vi "find readout time.vi"(8 "error in (no error)":errorcluster, 11 "Simulated_CCD_Camera in":refnum<class "Sim_Ixon_Ultra.lvclass">) -> (0 "error out":errorcluster, 3 "Simulated_CCD_Camera out":refnum<class "Sim_Ixon_Ultra.lvclass">)   [LabVIEW 2018, in "Sim_Ixon_Ultra.lvclass"]
doc: "Find the readout time as a function of the operation mode of the CCD.\n\nThis value is used to determine the minimum exposure time allowed by ACS, that is the readout time plus 10 % of this value. This procedure is related to the functioning of the frame transfer mode of the CCD and it prevents the misuse of the exposure time."
uses:
  Sim_Ixon_Ultra.lvclass
  C:/Users/Denis/Desktop/S4ACS/S4ACS/Sim_CCD/Sim_CCD.lvclass
  Sim_Ixon_Ultra.lvclass/Sim_Ixon_Ultra.ctl
  <vilib>/Utility/file.llb/Read Delimited Spreadsheet (DBL).vi
  Sim_CCD/Sim_CCD.lvclass
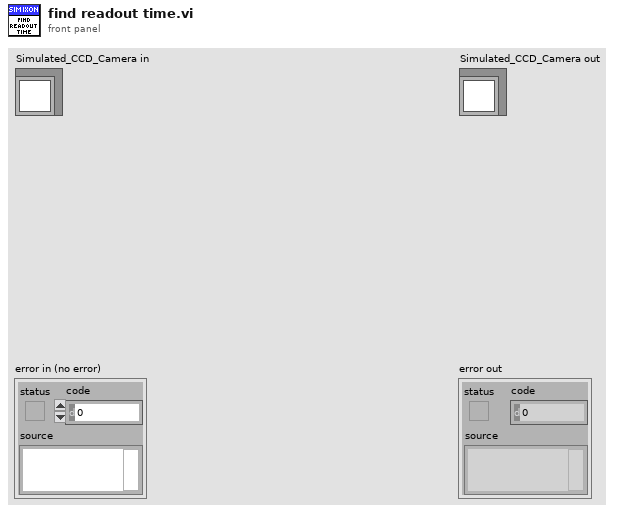
[diagram p1: front panel]
types:
  T1 = cluster{"PREAMP":u16, "READOUT_RATE":u16, "VERTICAL_SHIFT_SPEED":u16, "READ_MODE":u16, "VERTICAL_CLOCK_VOLTAGE":u16, "ACQUISITION_MODE":u16, "AD_CHANNEL":u16, "SHUTTER_TTL":u16, "SHUTTER_OPENING_TIME":u16, "SHUTTER_CLOSING_TIME":u16, "SHUTTER_MODE":u16, "TRIGGER_MODE":u16, "VBIN":u16, "INITIAL_LINE":u16, "INITIAL_COLUMN":u16, "FINAL_LINE":u16, "FINAL_COLUMN":u16, "HBIN":u16}
  T2 = typedef "LVDateTimeRec.ctl" = cluster{"fractional second":dbl, "second":i32, "minute":i32, "hour":i32, "day of month":i32, "month":i32, "year":i32, "day of week":i32, "day of year":i32, "DST":i32}
  T3 = cluster{"Time Acq Started":u32, "Image delay":u64, "Last update - CCD config":timestamp, "SYSTEMTIME":T2, "Readout time":dbl, "Time acq finished":u32, "effective exptime":dbl}
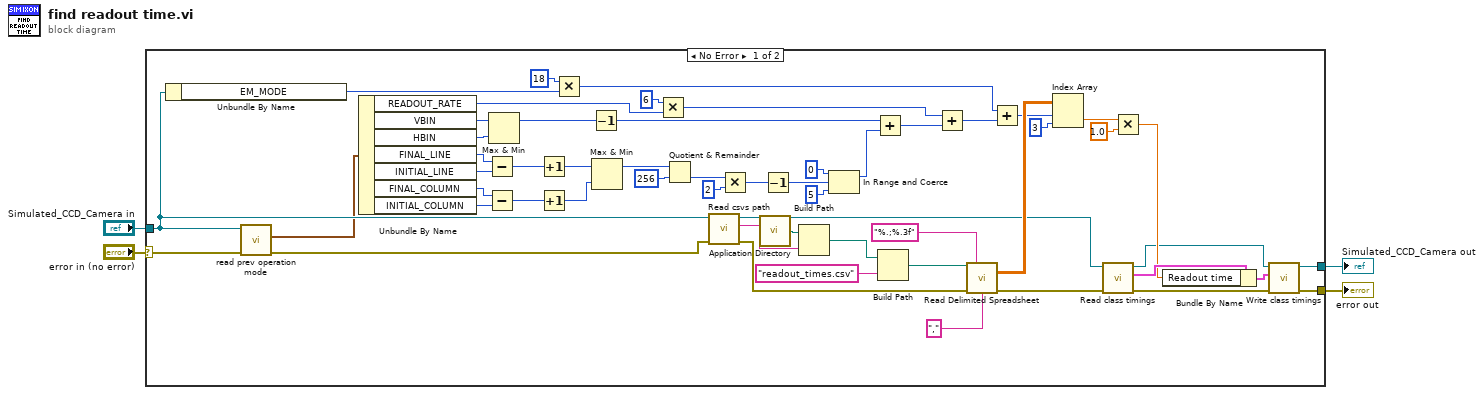
[diagram p0: block diagram]
diagram:
  n1 = case shown="No Error" "error in (no error)" {
    selector: "error in (no error)" -> [w7 w61]
    tunnel: [w19 w61] -> w3
    tunnel: [w21 w60] -> w1
    tunnel: "Simulated_CCD_Camera in" -> [w16 w60]
    frame No Error {
      n2 = Unbundle By Name(w16) -> ("EM_MODE"=w46:u16)
      n3 = call "read prev operation mode.vi"("error in (no error)"=w7, "Simulated_CCD_Camera in"=w16) -> ("error out"=w6:errorcluster, "prev operation mode"=w15:T1)  [unwired: 7 in, 1 out]
      n4 = Unbundle By Name(w15) -> ("READOUT_RATE"=w14:u16, "VBIN"=w13:u16, "HBIN"=w12:u16, "FINAL_LINE"=w11:u16, "INITIAL_LINE"=w10:u16, "FINAL_COLUMN"=w9:u16, "INITIAL_COLUMN"=w8:u16)
      n5 = Subtract(x=w11, y=w10) -> (x-y=w57:u16)
      n6 = Subtract(x=w9, y=w8) -> (x-y=w56:u16)
      n7 = Max & Min(x=w13, y=w12) -> (max(x,y)=w51:u16)  [unwired: 1 out]
      n8 = Increment(x=w57) -> (x+1=w55:u16)
      n9 = Increment(x=w56) -> (x+1=w54:u16)
      n10 = Multiply(x=u16 18, y=w46) -> (x*y=w43:u16)
      n11 = Decrement(x=w51) -> (x-1=w50:u16)
      n12 = Max & Min(x=w55, y=w54) -> (max(x,y)=w52:u16)  [unwired: 1 out]
      n13 = Multiply(x=u16 6, y=w14) -> (x*y=w47:u16)
      n14 = Quotient & Remainder(x=w52, y=u16 256) -> (floor(x/y)=w37:u16)  [unwired: 1 out]
      n15 = call "Read csvs path.vi"("error in (no error)"=w6, "Simulated Camera in"=w16) -> ("error out"=w26:errorcluster, "csvs path"=w5:string, "Simulated Camera out"=w18:refnum<class "Sim_Ixon_Ultra.lvclass">)  [unwired: 7 in]
      n16 = Multiply(x=w37, y=u16 2 ("x")) -> (x*y=w38:u16)
      n17 = call <vilib>:"Application Directory.vi"() -> ("Application Directory"=w58:path)
      n18 = Decrement(x=w38) -> (x-1=w36:u16)
      n19 = Build Path(base path=w58, name or relative path=w5) -> (appended path=w30:path)
      n20 = In Range and Coerce(upper limit=u16 0, x=w36, lower limit=u16 5 ("upper limit")) -> (coerced(x)=w33:u16)  [unwired: 1 out]
      n21 = Add(x=w50, y=w33) -> (x+y=w48:u16)
      n22 = Build Path(base path=w30, name or relative path="readout_times.csv") -> (appended path=w29:path)
      n23 = Add(x=w47, y=w48) -> (x+y=w44:u16)
      n24 = call-poly <vilib>:"Read Delimited Spreadsheet.vi"("file path (dialog if empty)"=w29, "format (%.3f)"="%.;%.3f", "error in (no error)"=w26, "delimiter (\\t)"="," ("delimiter (\\t)")) -> ("all rows"=w42:dbl[][], "error out"=w20:errorcluster)  [unwired: 6 in, 4 out]
      n25 = Add(x=w43, y=w44) -> (x+y=w40:u16)
      n26 = Index Array(array=w42, index (row)=w40, index (col)=3 ("disabled index (col)")) -> (element=w32:dbl)
      n27 = call "Read class timings.vi"("error in (no error)"=w20, "Simulated Camera in"=w18) -> ("error out"=w17:errorcluster, "class timings"=w25:T3, "Simulated Camera out"=w22:refnum<class "Sim_Ixon_Ultra.lvclass">)  [unwired: 7 in]
      n28 = Multiply(x=w32, y=1.0) -> (x*y=w23:dbl)
      n29 = Bundle By Name(cluster=w25, "Readout time"=w23) -> (w24:T3)
      n30 = call "Write class timings.vi"("error in (no error)"=w17, "class timings"=w24, "Simulated Camera in"=w22) -> ("error out"=w19:errorcluster, "Simulated Camera out"=w21:refnum<class "Sim_Ixon_Ultra.lvclass">)  [unwired: 7 in]
    }
    frame Error {
    }
  }
  "error out" <- w3
  "Simulated_CCD_Camera out" <- w1
